vi "AlarmSoundLoop.vi"(8 "Error In":errorcluster, 10 "ABLE Configuration":T1, 11 "Sound Data":refnum<notifier>) -> (0 "Error Out":errorcluster)   [LabVIEW 2012]
doc: "This VIs plays alarm sounds based on the activation of alarms."
uses:
  ABLEConfiguration.ctl
  DisplayConfiguration.ctl
  FolderConfiguration.ctl
  AlarmsConfiguration.ctl
  Keithley6485Configuration.ctl
  Keithley6482Configuration.ctl
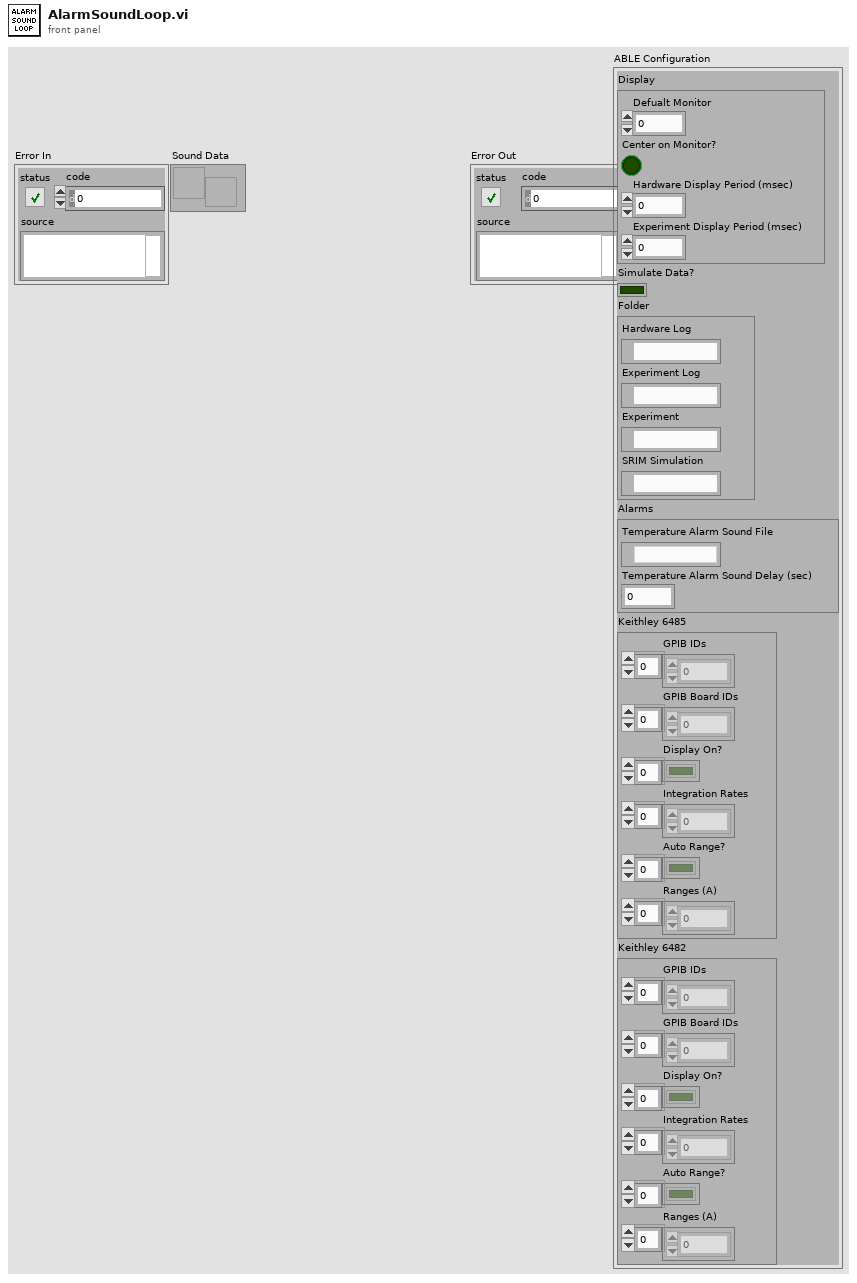
[diagram p1: front panel]
types:
  T1 = typedef "ABLEConfiguration.ctl" = cluster{"Display":T2, "Simulate Data?":bool, "Folder":T3, "Alarms":T4, "Keithley 6485":T5, "Keithley 6482":T6}
  T2 = typedef "DisplayConfiguration.ctl" = cluster{"Defualt Monitor":u16, "Center on Monitor?":bool, "Hardware Display Period (msec)":u32, "Experiment Display Period (msec)":u32}
  T3 = typedef "FolderConfiguration.ctl" = cluster{"Hardware Log":path, "Experiment Log":path, "Experiment":path, "SRIM Simulation":path}
  T4 = typedef "AlarmsConfiguration.ctl" = cluster{"Temperature Alarm Sound File":path, "Temperature Alarm Sound Delay (sec)":dbl}
  T5 = typedef "Keithley6485Configuration.ctl" = cluster{"GPIB IDs":u8[], "GPIB Board IDs":u8[], "Display On?":bool[], "Integration Rates":dbl[], "Auto Range?":bool[], "Ranges (A)":dbl[]}
  T6 = typedef "Keithley6482Configuration.ctl" = cluster{"GPIB IDs":u8[], "GPIB Board IDs":u8[], "Display On?":bool[], "Integration Rates":dbl[], "Auto Range?":bool[], "Ranges (A)":dbl[]}
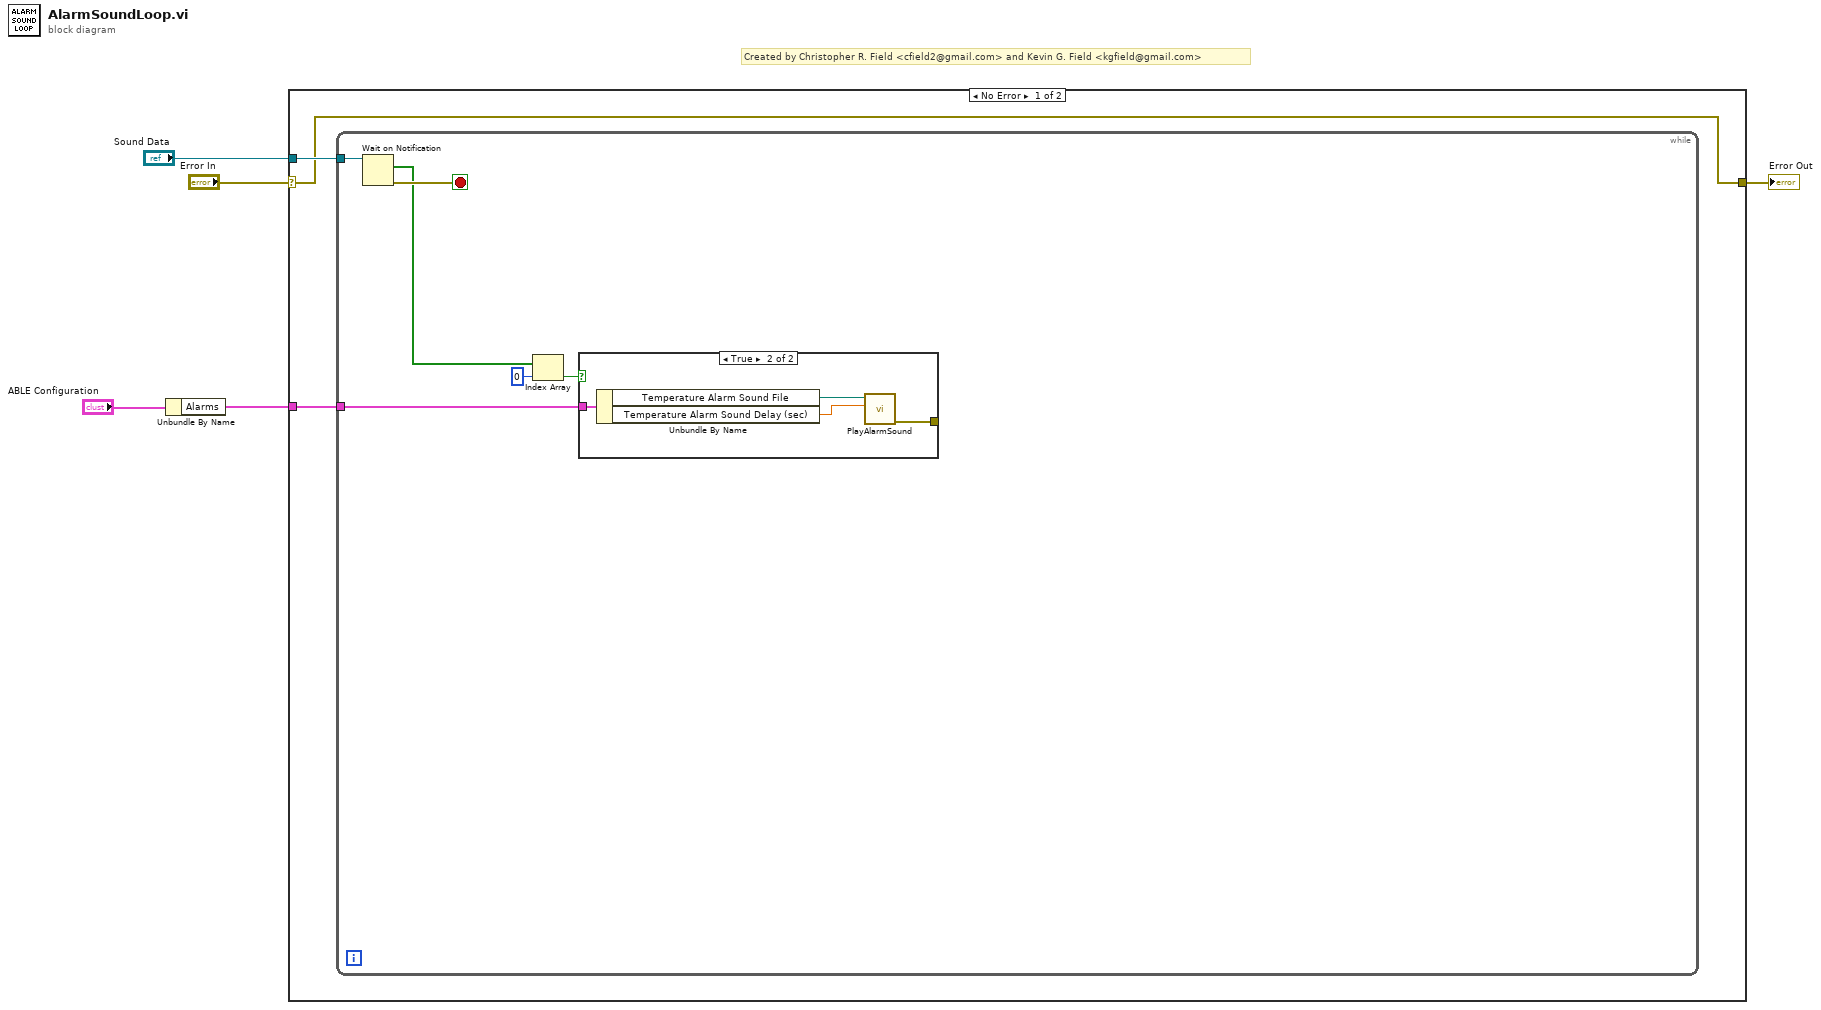
[diagram p0: block diagram]
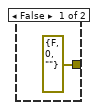
[diagram p2: hidden frame]
diagram:
  # "Created by Christopher R. Field <cfield2@gmail.com> and Kevin G. Field <kgfield@gmail.com>"
  n1 = Unbundle By Name("ABLE Configuration") -> ("Alarms"=w1:T4)
  n2 = case shown="No Error" "Error In" {
    selector: "Error In" -> [w6 w20]
    tunnel: [w6 w20] -> w4
    tunnel: "Sound Data" -> [w8 _]
    tunnel: w1 -> [w7 _]
    frame No Error {
      n3 = while {
        tunnel: w8 -> [w14]
        tunnel: w7 -> [w9]
        stop <- w11 stop-if-true
        n4 = Wait on Notification(notifier=w14) -> (notification=w10:bool[], error out=w11:errorcluster)  [unwired: 3 in, 2 out]
        n5 = Index Array(array=w10, index=0) -> (element=w12:bool)
        n6 = case shown="True" w12 {
          tunnel: w9 -> [_ w19]
          tunnel: [errorcluster {"status"=FALSE, "code"=0, "source"=""} ("Error Out") w16] -> _
          frame False {
          }
          frame True {
            n7 = Unbundle By Name(w19) -> ("Temperature Alarm Sound File"=w18:path, "Temperature Alarm Sound Delay (sec)"=w17:dbl)
            n8 = call "PlayAlarmSound.vi"("Alarm Sound Delay (sec)"=w17, "Alarm Sound File Path"=w18) -> ("Error Out"=w16:errorcluster)  [unwired: 9 in]
          }
        }
      }
    }
    frame Error {
    }
  }
  "Error Out" <- w4
